vi "Test WS Local Echo Server.vi"(8 "error in (no error)":errorcluster, 11 "TestCase in":refnum<class "Test WebSockets Server.lvclass">) -> (0 "error out":errorcluster, 3 "TestCase out":refnum<class "Test WebSockets Server.lvclass">)   [LabVIEW 2013, in "Test WebSockets Server.lvclass"]
uses:
  Test WebSockets Server.lvclass
  <vilib>/addons/_JKI Toolkits/VI Tester/TestCase.llb/TestCase.lvclass
  WebSockets/WebSockets.lvlib
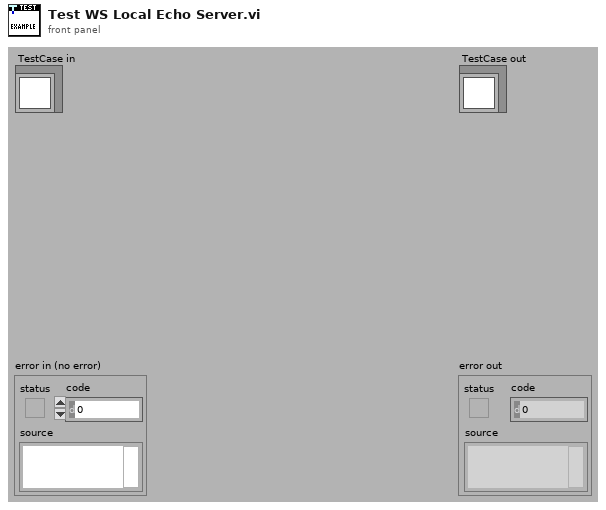
[diagram p1: front panel]
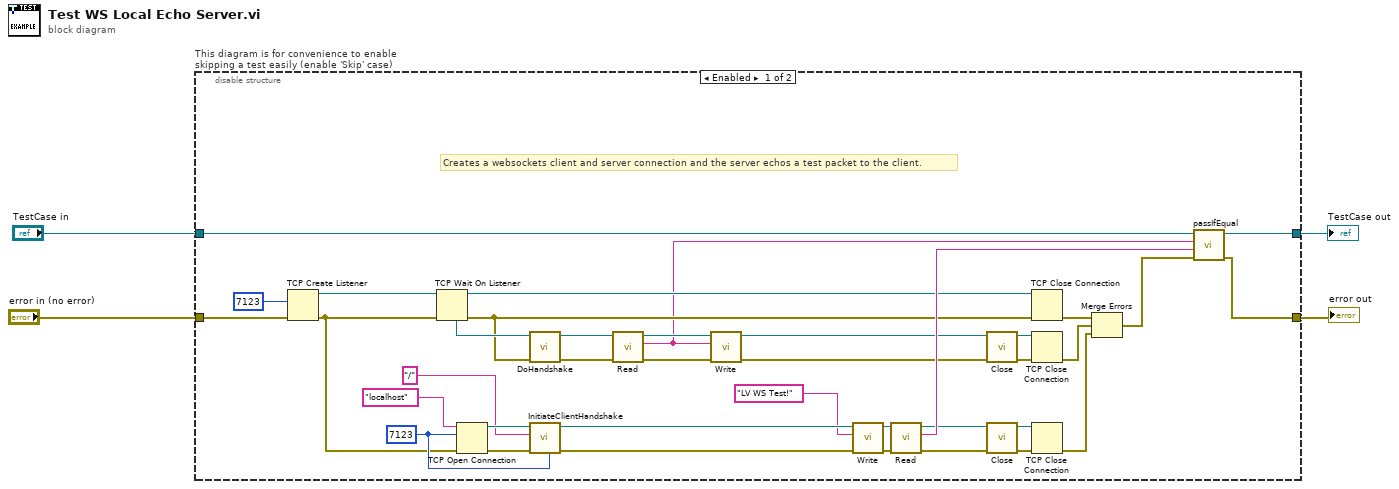
[diagram p0: block diagram]
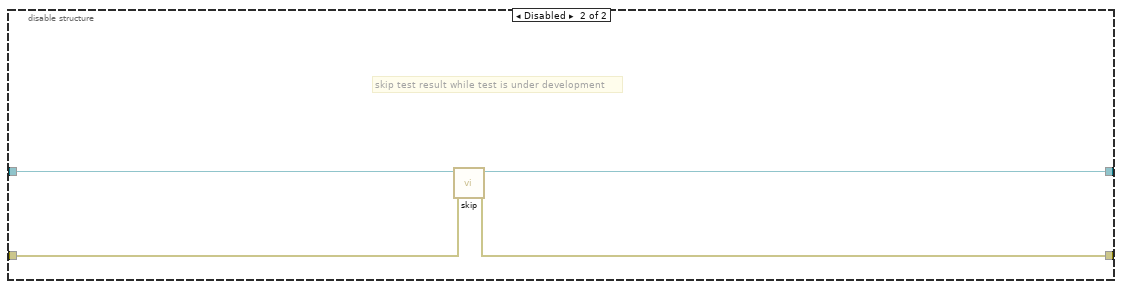
[diagram p2: hidden frame]
diagram:
  n1 = disable-structure "This diagram is for convenience to enable skipping a test easily (enable 'Skip' case)" shown="Enabled" {
    disable-tunnel: "TestCase in" -> [w33 w46]
    disable-tunnel: [w32 w44] -> w1
    disable-tunnel: [w31 w45] -> w3
    disable-tunnel: "error in (no error)" -> [w29 w43]
    frame Enabled {
      w36 = u16 7123 ("remote port or service name")
      # "Creates a websockets client and server connection and the server echos a test packet to the client."
      n2 = TCP Create Listener(8:w29, 10:u16 7123 ("port")) -> (0:w22:errorcluster, 3:w21:refnum<k5>)  [unwired: 3 in, 1 out]
      n3 = TCP Wait On Listener(8:w22, 11:w21) -> (0:w16:errorcluster, 3:w17:refnum<k5>, 4:w20:refnum<k5>)  [unwired: 2 in, 2 out]
      n4 = TCP Open Connection(address="localhost", remote port or service name=w36, error in (no error)=w22) -> (connection ID=w42:refnum<k5>, error out=w41:errorcluster)  [unwired: 2 in]
      n5 = call "DoHandshake.vi"("error in (no error)"=w16, "WebSocket Connection in"=w20) -> ("error out"=w28:errorcluster, "WebSocket Connection out"=w25:refnum<k5>)  [unwired: 6 in, 2 out]
      n6 = call "InitiateClientHandshake.vi"("remote port or service name"=w36, "error in (no error)"=w41, "request URI ('/')"="/", "WebSocket Connection in"=w42) -> ("error out"=w40:errorcluster, "WebSocket Connection out"=w39:refnum<k5>)  [unwired: 5 in, 1 out]
      n7 = call "Read.vi"("error in (no error)"=w28, "WebSocket Connection in"=w25) -> ("error out"=w27:errorcluster, "Data"=w5:string, "WebSocket Connection out"=w26:refnum<k5>)  [unwired: 5 in, 2 out]
      n8 = call "Write.vi"("error in (no error)"=w27, "Data"=w5, "WebSocket Connection in"=w26) -> ("error out"=w19:errorcluster, "WebSocket Connection out"=w18:refnum<k5>)  [unwired: 7 in]
      n9 = call "Write.vi"("error in (no error)"=w40, "Data"="LV WS Test!", "WebSocket Connection in"=w39) -> ("error out"=w38:errorcluster, "WebSocket Connection out"=w37:refnum<k5>)  [unwired: 7 in]
      n10 = call "Read.vi"("error in (no error)"=w38, "WebSocket Connection in"=w37) -> ("error out"=w14:errorcluster, "Data"=w24:string, "WebSocket Connection out"=w13:refnum<k5>)  [unwired: 5 in, 2 out]
      n11 = call "Close.vi"("error in (no error)"=w19, "WebSocket Connection in"=w18) -> ("error out"=w15:errorcluster, "WebSocket Connection in"=w10:refnum<k5>)  [unwired: 8 in]
      n12 = call "Close.vi"("error in (no error)"=w14, "WebSocket Connection in"=w13) -> ("error out"=w11:errorcluster, "WebSocket Connection in"=w12:refnum<k5>)  [unwired: 8 in]
      n13 = TCP Close Connection(connection ID=w17, error in (no error)=w16) -> (error out=w9:errorcluster)  [unwired: 1 in, 1 out]
      n14 = TCP Close Connection(connection ID=w10, error in (no error)=w15) -> (error out=w8:errorcluster)  [unwired: 1 in, 1 out]
      n15 = TCP Close Connection(connection ID=w12, error in (no error)=w11) -> (error out=w7:errorcluster)  [unwired: 1 in, 1 out]
      n16 = Merge Errors(w9, w8, w7) -> (w6:errorcluster)
      n17 = call-dynamic "passIfEqual.vi"("error in (no error)"=w6, "y"=w24, "x"=w5, "TestCase in"=w33) -> ("error out"=w31:errorcluster, "TestCase out"=w32:refnum<class "Test WebSockets Server.lvclass">)  [unwired: 6 in]
    }
    frame Disabled {
      # "skip test result while test is under development"
      n18 = call <vilib>:"skip.vi"("error in (no error)"=w43, "TestCase in"=w46) -> ("error out"=w45:errorcluster, "TestCase out"=w44:refnum<class "Test WebSockets Server.lvclass">)  [unwired: 8 in]
    }
  }
  "error out" <- w3
  "TestCase out" <- w1
